vi "Configure TS Relays.vi"(8 "error in":errorcluster, 11 "DeepU Test Stand in":refnum<class "DeepU Test Stand.lvclass">) -> (0 "error out":errorcluster, 3 "DeepU Test Stand out":refnum<class "DeepU Test Stand.lvclass">)   [LabVIEW 2019, in "Test Stands.lvlib" / "DeepU Test Stand.lvclass"]
uses:
  DeepU Test Stand.lvclass
  DeepU Test Stand.lvclass/DeepU Test Stand.ctl
  <vilib>/DAQmx/create/channels.llb/DAQmx Create Channel (DO-Digital Output).vi
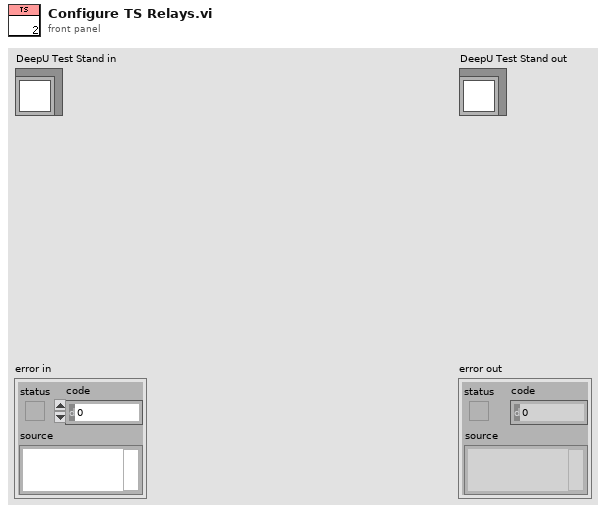
[diagram p1: front panel]
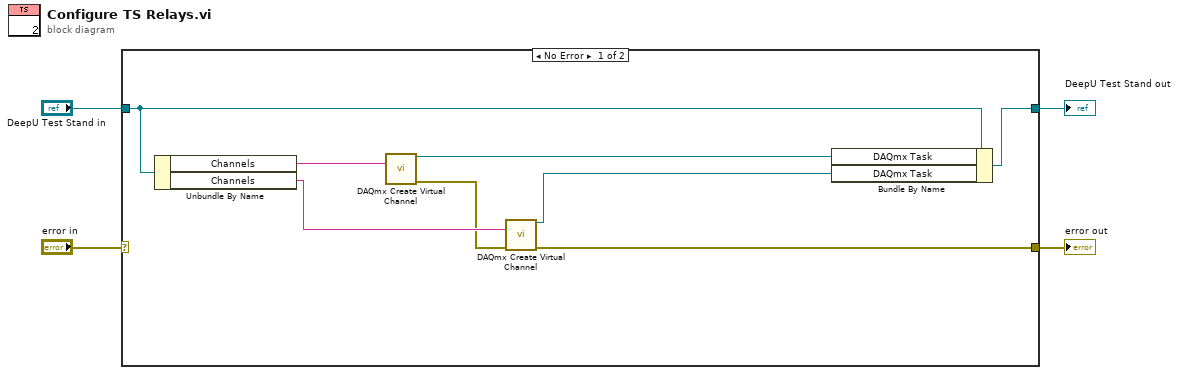
[diagram p0: block diagram]
diagram:
  n1 = case shown="No Error" "error in" {
    selector: "error in" -> [_ w14]
    tunnel: [w6 w14] -> w3
    tunnel: [w11 w13] -> w1
    tunnel: "DeepU Test Stand in" -> [w12 w13]
    frame No Error {
      n2 = Unbundle By Name(w12) -> ("Channels"=w10:string, "Channels"=w9:string)
      n3 = call-poly <vilib>:"DAQmx Create Virtual Channel.vi"("lines"=w10) -> ("task out"=w8:refnum<k21>, "error out"=w7:errorcluster)  [unwired: 13 in]
      n4 = call-poly <vilib>:"DAQmx Create Virtual Channel.vi"("lines"=w9, "error in"=w7) -> ("task out"=w5:refnum<k21>, "error out"=w6:errorcluster)  [unwired: 12 in]
      n5 = Bundle By Name(cluster=w12, "DAQmx Task"=w8, "DAQmx Task"=w5) -> (w11:refnum<class "DeepU Test Stand.lvclass">)
    }
    frame Error {
    }
  }
  "error out" <- w3
  "DeepU Test Stand out" <- w1
